vi "Fase 3_Grupo 1.vi"() -> ()   [LabVIEW 2020]
panel:
  out "Enfriamiento":bool
  out "Calentamiento":bool
  out "Fin":bool
  out "Inicio":bool
  out "Horno":bool
  out "Ventilador":bool
  out "Temperat":dbl(slide) scale=0.0..150.0 scale format="%#.2g"
  in  "Abortar":bool
  in  "Parada 2":bool
  in  "Marcha 2":bool
  out "Enfriar":bool
  out "Calentar":bool
  out "Control Temperatura":dynamicdata(graph)
  in  "Temp Inferior":dbl
  in  "Temp Superior":dbl
  in  "Temp Proceso":dbl
  # "Torrefacción"
  # "Silo triturado"
  # "Dídier Javier Ramírez Henao"
  # "Calentamiento"
  # "Enfriamiento"
  # "Pulsadores de mando"
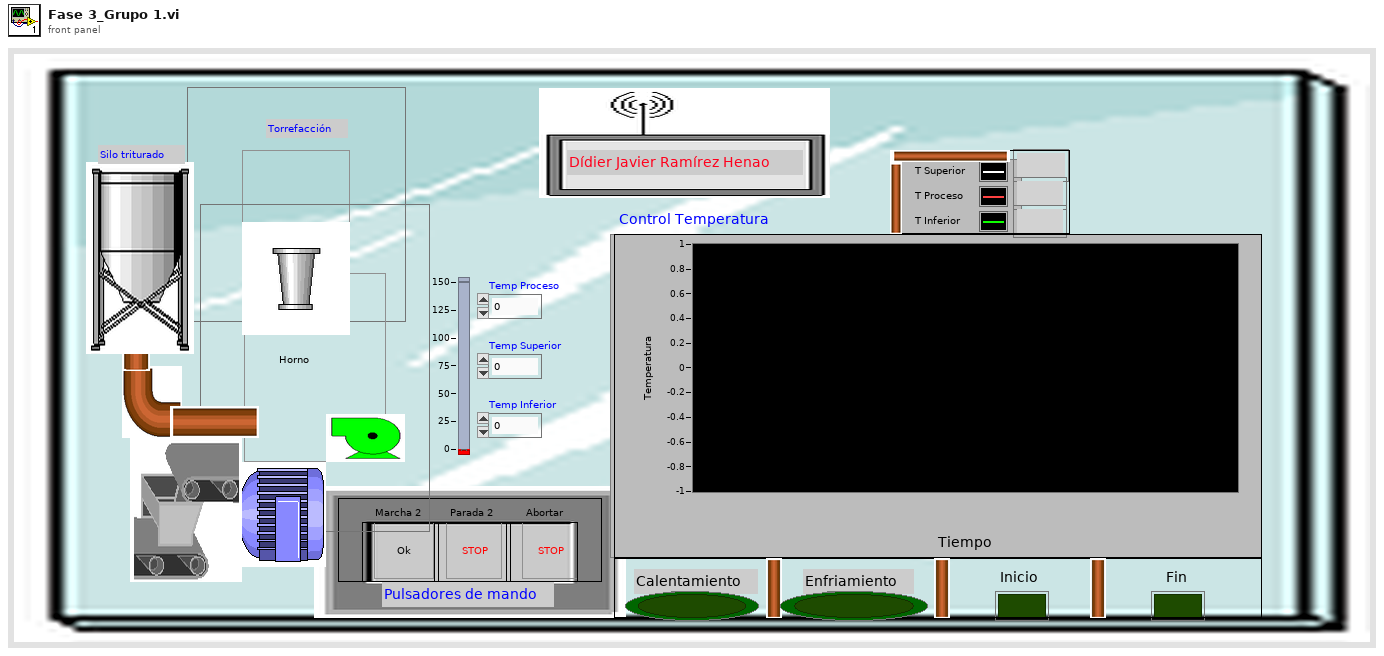
[diagram p1: front panel]
types:
  T1 = enum16{"INICIO", "CALENTAR", "ENFRIAR", "PARO", "ABORTAR", "FIN"}
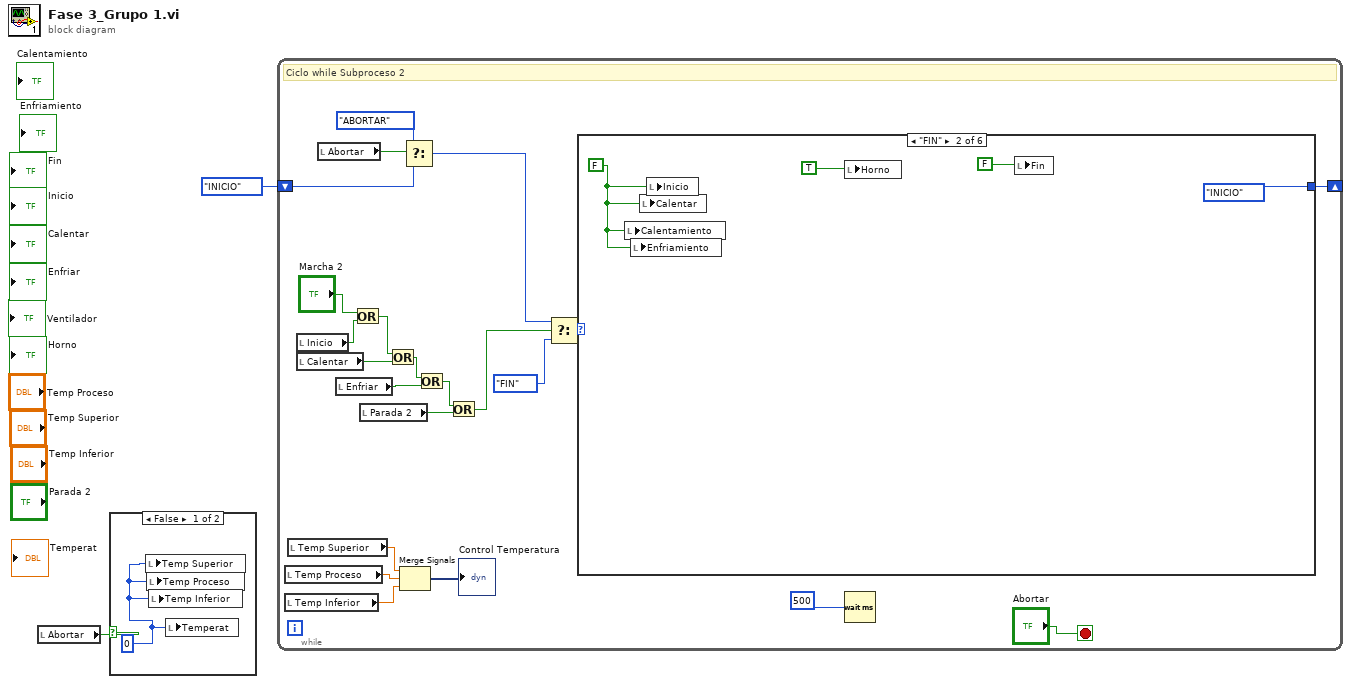
[diagram p0: block diagram]
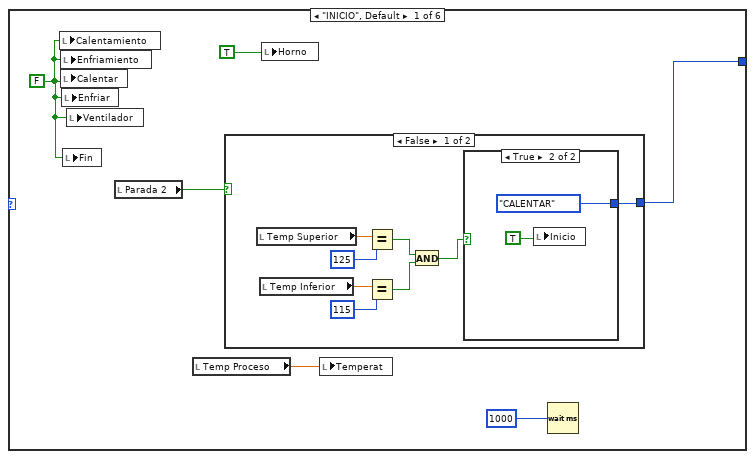
[diagram p3: hidden frame]
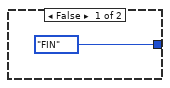
[diagram p4: hidden frame]
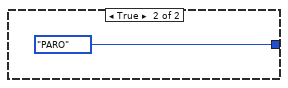
[diagram p5: hidden frame]
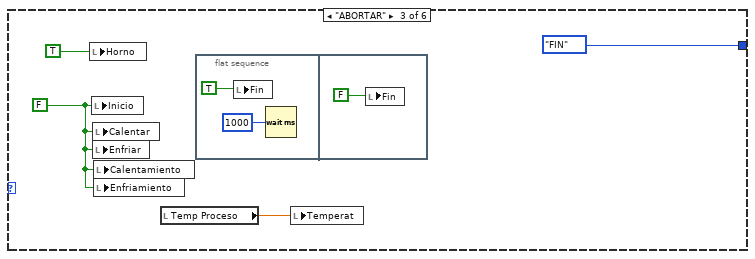
[diagram p6: hidden frame]
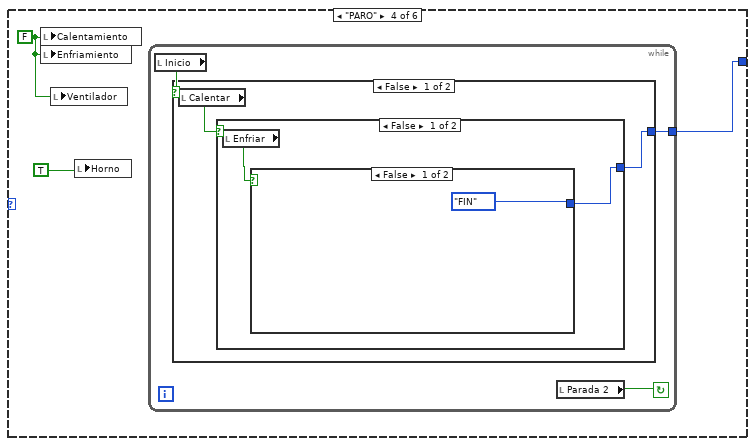
[diagram p7: hidden frame]
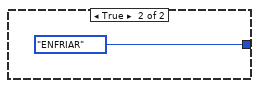
[diagram p8: hidden frame]
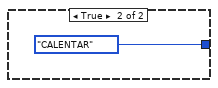
[diagram p9: hidden frame]
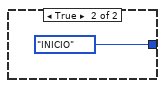
[diagram p10: hidden frame]
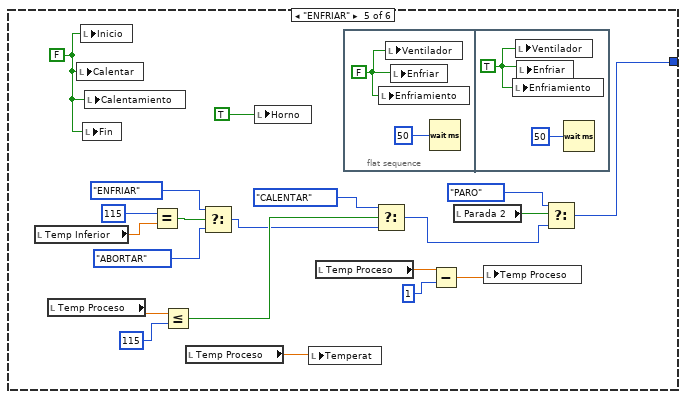
[diagram p11: hidden frame]
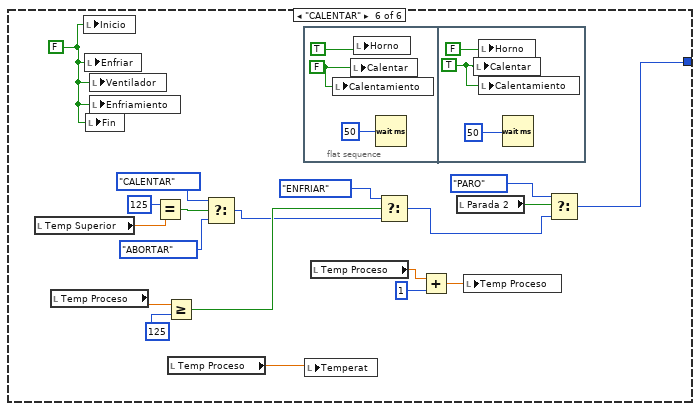
[diagram p12: hidden frame]
diagram:
  n1 = local read "Abortar"() -> (w1:bool)
  n2 = case shown="False" w1 {
    frame False {
      w3 = 0
      n3 = local write "Temp Superior"(w3) -> ()
      n4 = local write "Temp Proceso"(w3) -> ()
      n5 = local write "Temp Inferior"(w3) -> ()
      n6 = local write "Temperat"(w3) -> ()
    }
    frame True {
    }
  }
  n7 = while {
    shift-right: [w11] -> _
    shift-left: T1."INICIO" -> [w24]
    stop <- "Abortar" stop-if-true
    # "Ciclo while Subproceso 2"
    n8 = local read "Temp Proceso"() -> (w6:dbl)
    n9 = local read "Temp Inferior"() -> (w5:dbl)
    n10 = local read "Temp Superior"() -> (w7:dbl)
    n11 = local read "Inicio"() -> (w20:bool)
    n12 = local read "Calentar"() -> (w18:bool)
    n13 = local read "Abortar"() -> (w10:bool)
    n14 = local read "Enfriar"() -> (w16:bool)
    n15 = Or(x="Marcha 2", y=w20) -> (x .or. y?=w19:bool)
    n16 = local read "Parada 2"() -> (w14:bool)
    n17 = Or(x=w19, y=w18) -> (x .or. y?=w17:bool)
    n18 = Merge Signals(w7, w6, w5) -> (→"Control Temperatura":dynamicdata)
    n19 = Select(t=T1."ABORTAR", s=w10, f=w24) -> (s? t:f=w22:T1)
    n20 = Or(x=w17, y=w16) -> (x .or. y?=w15:bool)
    n21 = Or(x=w15, y=w14) -> (x .or. y?=w13:bool)
    n22 = Select(t=w22, s=w13, f=T1."FIN") -> (s? t:f=w21:T1)
    n23 = case shown="\"FIN\"" w21 {
      tunnel: [w30 T1."INICIO" T1."FIN" w57 w75 w102] -> w11
      frame "INICIO", Default {
        w27 = FALSE
        n24 = local write "Calentamiento"(w27) -> ()
        n25 = local write "Enfriamiento"(w27) -> ()
        n26 = local write "Calentar"(w27) -> ()
        n27 = local write "Enfriar"(w27) -> ()
        n28 = local write "Fin"(w27) -> ()
        n29 = local write "Ventilador"(w27) -> ()
        n30 = local read "Parada 2"() -> (w31:bool)
        n31 = local read "Temp Proceso"() -> (w29:dbl)
        n32 = case shown="False" w31 {
          tunnel: [w37 T1."PARO"] -> w30
          frame False {
            n33 = local read "Temp Superior"() -> (w39:dbl)
            n34 = local read "Temp Inferior"() -> (w35:dbl)
            n35 = Equal?(x=w39, y=125) -> (x = y?=w34:bool)
            n36 = Equal?(x=w35, y=115) -> (x = y?=w32:bool)
            n37 = And(x=w34, y=w32) -> (x .and. y?=w33:bool)
            n38 = case shown="True" w33 {
              tunnel: [T1."FIN" T1."CALENTAR"] -> w37
              frame False {
              }
              frame True {
                n39 = local write "Inicio"(TRUE) -> ()
              }
            }
          }
          frame True {
          }
        }
        n40 = local write "Horno"(TRUE) -> ()
        n41 = local write "Temperat"(w29) -> ()
        n42 = Wait (ms)(milliseconds to wait=1000) -> ()  [unwired: 1 out]
      }
      frame "FIN" {
        w44 = FALSE
        n43 = local write "Calentamiento"(w44) -> ()
        n44 = local write "Enfriamiento"(w44) -> ()
        n45 = local write "Calentar"(w44) -> ()
        n46 = local write "Inicio"(w44) -> ()
        n47 = local write "Horno"(TRUE) -> ()
        n48 = local write "Fin"(FALSE) -> ()
      }
      frame "ABORTAR" {
        w49 = FALSE
        n49 = local write "Horno"(TRUE) -> ()
        n50 = local write "Inicio"(w49) -> ()
        n51 = local write "Calentar"(w49) -> ()
        n52 = local write "Enfriar"(w49) -> ()
        n53 = local write "Calentamiento"(w49) -> ()
        n54 = local write "Enfriamiento"(w49) -> ()
        n55 = local read "Temp Proceso"() -> (w50:dbl)
        n56 = flat-sequence {
          frame #0 {
            n57 = local write "Fin"(TRUE) -> ()
            n58 = Wait (ms)(milliseconds to wait=1000) -> ()  [unwired: 1 out]
          }
          frame #1 {
            n59 = local write "Fin"(FALSE) -> ()
          }
        }
        n60 = local write "Temperat"(w50) -> ()
      }
      frame "PARO" {
        w56 = FALSE
        n61 = local write "Calentamiento"(w56) -> ()
        n62 = local write "Enfriamiento"(w56) -> ()
        n63 = local write "Ventilador"(w56) -> ()
        n64 = local write "Horno"(TRUE) -> ()
        n65 = while {
          tunnel: [w59] -> w57
          stop <- w60 continue-if-true
          n66 = local read "Inicio"() -> (w58:bool)
          n67 = case shown="False" w58 {
            tunnel: [w61 T1."INICIO"] -> w59
            frame False {
              n68 = local read "Calentar"() -> (w62:bool)
              n69 = case shown="False" w62 {
                tunnel: [w64 T1."CALENTAR"] -> w61
                frame False {
                  n70 = local read "Enfriar"() -> (w63:bool)
                  n71 = case shown="False" w63 {
                    tunnel: [T1."FIN" T1."ENFRIAR"] -> w64
                    frame False {
                    }
                    frame True {
                    }
                  }
                }
                frame True {
                }
              }
            }
            frame True {
            }
          }
          n72 = local read "Parada 2"() -> (w60:bool)
        }
      }
      frame "ENFRIAR" {
        w69 = FALSE
        n73 = local read "Temp Inferior"() -> (w88:dbl)
        n74 = local read "Temp Proceso"() -> (w83:dbl)
        n75 = local write "Calentar"(w69) -> ()
        n76 = local write "Inicio"(w69) -> ()
        n77 = local write "Fin"(w69) -> ()
        n78 = local write "Calentamiento"(w69) -> ()
        n79 = Equal?(x=115, y=w88) -> (x = y?=w87:bool)
        n80 = Less Or Equal?(x=w83, y=115) -> (x <= y?=w86:bool)
        n81 = local read "Temp Proceso"() -> (w74:dbl)
        n82 = Select(t=T1."ENFRIAR", s=w87, f=T1."ABORTAR") -> (s? t:f=w85:T1)
        n83 = local write "Horno"(TRUE) -> ()
        n84 = local write "Temperat"(w74) -> ()
        n85 = local read "Temp Proceso"() -> (w73:dbl)
        n86 = flat-sequence {
          frame #0 {
            w89 = FALSE
            n87 = local write "Enfriamiento"(w89) -> ()
            n88 = local write "Ventilador"(w89) -> ()
            n89 = local write "Enfriar"(w89) -> ()
            n90 = Wait (ms)(milliseconds to wait=50) -> ()  [unwired: 1 out]
          }
          frame #1 {
            w91 = TRUE
            n91 = local write "Enfriamiento"(w91) -> ()
            n92 = local write "Ventilador"(w91) -> ()
            n93 = local write "Enfriar"(w91) -> ()
            n94 = Wait (ms)(milliseconds to wait=50) -> ()  [unwired: 1 out]
          }
        }
        n95 = Select(t=T1."CALENTAR", s=w86, f=w85) -> (s? t:f=w82:T1)
        n96 = Subtract(x=w73, y=1) -> (x-y=w71:dbl)
        n97 = local read "Parada 2"() -> (w84:bool)
        n98 = local write "Temp Proceso"(w71) -> ()
        n99 = Select(t=T1."PARO", s=w84, f=w82) -> (s? t:f=w75:T1)
      }
      frame "CALENTAR" {
        w93 = FALSE
        n100 = local read "Temp Superior"() -> (w110:dbl)
        n101 = local read "Temp Proceso"() -> (w100:dbl)
        n102 = local write "Inicio"(w93) -> ()
        n103 = local write "Enfriar"(w93) -> ()
        n104 = local write "Fin"(w93) -> ()
        n105 = local write "Ventilador"(w93) -> ()
        n106 = local write "Enfriamiento"(w93) -> ()
        n107 = Equal?(x=125, y=w110) -> (x = y?=w109:bool)
        n108 = Greater Or Equal?(x=w100, y=125) -> (x >= y?=w106:bool)
        n109 = local read "Temp Proceso"() -> (w97:dbl)
        n110 = Select(t=T1."CALENTAR", s=w109, f=T1."ABORTAR") -> (s? t:f=w105:T1)
        n111 = flat-sequence {
          frame #0 {
            w112 = FALSE
            n112 = local write "Calentamiento"(w112) -> ()
            n113 = local write "Calentar"(w112) -> ()
            n114 = local write "Horno"(TRUE) -> ()
            n115 = Wait (ms)(milliseconds to wait=50) -> ()  [unwired: 1 out]
          }
          frame #1 {
            w115 = TRUE
            n116 = local write "Calentar"(w115) -> ()
            n117 = local write "Horno"(FALSE) -> ()
            n118 = local write "Calentamiento"(w115) -> ()
            n119 = Wait (ms)(milliseconds to wait=50) -> ()  [unwired: 1 out]
          }
        }
        n120 = local write "Temperat"(w97) -> ()
        n121 = local read "Temp Proceso"() -> (w96:dbl)
        n122 = Select(t=T1."ENFRIAR", s=w106, f=w105) -> (s? t:f=w98:T1)
        n123 = Add(x=w96, y=1) -> (x+y=w94:dbl)
        n124 = local read "Parada 2"() -> (w103:bool)
        n125 = local write "Temp Proceso"(w94) -> ()
        n126 = Select(t=T1."PARO", s=w103, f=w98) -> (s? t:f=w102:T1)
      }
    }
    n127 = Wait (ms)(milliseconds to wait=500) -> ()  [unwired: 1 out]
  }
